vi "Close.vi"(8 "error in":errorcluster, 11 "IMAQdx Base Configure Strategy in":refnum<class "IMAQdx Base Configure Strategy.lvclass">) -> (0 "error out":errorcluster, 3 "IMAQdx Base Configure Strategy out":refnum<class "IMAQdx Base Configure Strategy.lvclass">)   [LabVIEW 2024, in "IMAQdx Base Configure Strategy.lvclass"]
uses:
  IMAQdx Base Configure Strategy.lvclass
  IMAQdx Base Configure Strategy.lvclass/IMAQdx Base Configure Strategy.ctl
  <vilib>/vision/driver/NI_Vision_Acquisition_Software.lvlib
  <vilib>/userDefined/High Color/IMAQdx.ctl
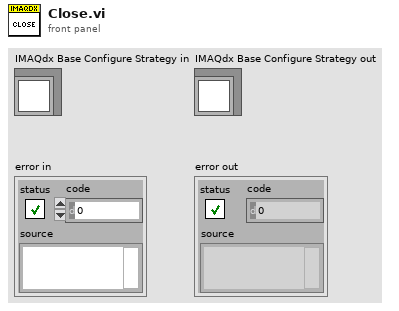
[diagram p1: front panel]
types:
  T1 = typedef "IMAQdx.ctl" = refnum<k21>
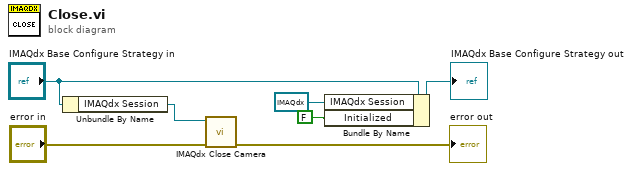
[diagram p0: block diagram]
diagram:
  n1 = Unbundle By Name("IMAQdx Base Configure Strategy in") -> ("IMAQdx Session"=w6:T1)
  n2 = call <vilib>:"IMAQdx Close Camera.vi"("error in"="error in", "Session In"=w6) -> ("error out"=→"error out":errorcluster)  [unwired: 9 in]
  n3 = Bundle By Name(cluster="IMAQdx Base Configure Strategy in", "IMAQdx Session"=T1 refnum, "Initialized"=FALSE) -> (→"IMAQdx Base Configure Strategy out":refnum<class "IMAQdx Base Configure Strategy.lvclass">)
